vi "test_MSS simulated daqmx do.vi"(8 "Error In":errorcluster) -> (0 "Error Out":errorcluster)   [LabVIEW 2023]
uses:
  Virtual DIO/Virt PWM Generator/Virt DAQmx PWM Generator.lvclass
  Measure and Stimulus Subsystems/Measure and Stimulus Subsystems.lvclass
panel:
  in  "Stop":bool
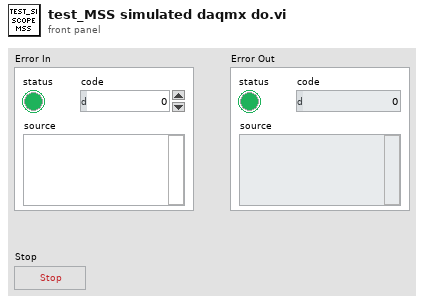
[diagram p1: front panel]
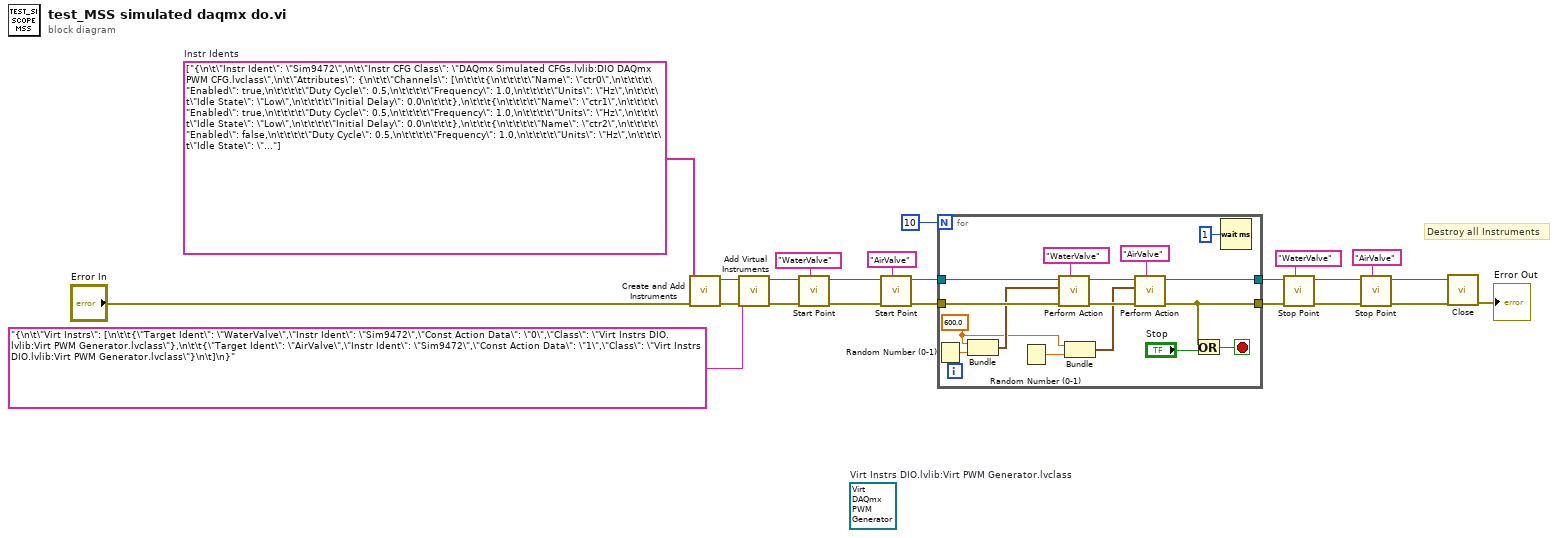
[diagram p0: block diagram]
diagram:
  (unwired) refnum<class "Virt DAQmx PWM Generator.lvclass"> refnum  # Virt Instrs DIO.lvlib:Virt PWM Generator.lvclass
  w19 = string[] ["{\n\t\"Instr Ident\": \"Sim9472\",\n\t\"Instr CFG Class\": \"DAQmx Simulated CFGs.lvlib:DIO DAQmx PWM CFG.lvclass\",\n\t\"Attributes\": {\n\t\t\"Channels\": [\n\t\t\t{\n\t\t\t\t\"Name\": \"ctr0\",\n\t\t\t\t\"Enabled\": true,\n\t\t\t\t\"Duty Cycle\": 0.5,\n\t\t\t\t\"Frequency\": 1.0,\n\t\t\t\t\"Units\": \"Hz\",\n\t\t\t\t\"Idle State\": \"Low\",\n\t\t\t\t\"Initial Delay\": 0.0\n\t\t\t},\n\t\t\t{\n\t\t\t\t\"Name\": \"ctr1\",\n\t\t\t\t\"Enabled\": true,\n\t\t\t\t\"Duty Cycle\": 0.5,\n\t\t\t\t\"Frequency\": 1.0,\n\t\t\t\t\"Units\": \"Hz\",\n\t\t\t\t\"Idle State\": \"Low\",\n\t\t\t\t\"Initial Delay\": 0.0\n\t\t\t},\n\t\t\t{\n\t\t\t\t\"Name\": \"ctr2\",\n\t\t\t\t\"Enabled\": false,\n\t\t\t\t\"Duty Cycle\": 0.5,\n\t\t\t\t\"Frequency\": 1.0,\n\t\t\t\t\"Units\": \"Hz\",\n\t\t\t\t\"Idle State\": \"Low\",\n\t\t\t\t\"Initial Delay\": 0.0\n\t\t\t},\n\t\t\t{\n\t\t\t\t\"Name\": \"ctr3\",\n\t\t\t\t\"Enabled\": false,\n\t\t\t\t\"Duty Cycle\": 0.5,\n\t\t\t\t\"Frequency\": 1.0,\n\t\t\t\t\"Units\": \"Hz\",\n\t\t\t\t\"Idle State\": \"Low\",\n\t\t\t\t\"Initial Delay\": 0.0\n\t\t\t}\n\t\t],\n\t\t\"Timing\": {\n\t\t\t\"Samples per Channel\": 1000,\n\t\t\t\"Sample Mode\": \"Continuous Samples\",\n\t\t\t\"Sample Rate\": 0.0,\n\t\t\t\"Sample Clock Source\": \"Implicit\",\n\t\t\t\"Active Edge\": \"Rising\"\n\t\t},\n\t\t\"Trigger\": {\n\t\t\t\"Trigger Type\": \"No Trigger\"\n\t\t}\n\t}\n}"]  # Instr Idents
  # "Destroy all Instruments"
  n1 = call "Create and Add Instruments.vi"("Error In"="Error In", "Physical Intr CFGs"=w19) -> ("Error Out"=w20:errorcluster, "MSS out"=w5:refnum<class "Measure and Stimulus Subsystems.lvclass">)  [unwired: 8 in]
  n2 = call "Add Virtual Instruments.vi"("error in"=w20, "<JSON CFG>"="{\n\t\"Virt Instrs\": [\n\t\t{\"Target Ident\": \"WaterValve\",\"Instr Ident\": \"Sim9472\",\"Const Action Data\": \"0\",\"Class\": \"Virt Instrs DIO.lvlib:Virt PWM Generator.lvclass\"},\n\t\t{\"Target Ident\": \"AirValve\",\"Instr Ident\": \"Sim9472\",\"Const Action Data\": \"1\",\"Class\": \"Virt Instrs DIO.lvlib:Virt PWM Generator.lvclass\"}\n\t]\n}", "MSS in"=w5) -> ("error out"=w6:errorcluster, "MSS out"=w4:refnum<class "Measure and Stimulus Subsystems.lvclass">)  [unwired: 7 in]
  n3 = call "Start Point.vi"("Point Ident"="WaterValve" ("Target Ident"), "error in"=w6, "MSS in"=w4) -> ("error out"=w18:errorcluster, "MSS out"=w16:refnum<class "Measure and Stimulus Subsystems.lvclass">)  [unwired: 7 in]
  n4 = call "Start Point.vi"("Point Ident"="AirValve" ("Target Ident"), "error in"=w18, "MSS in"=w16) -> ("error out"=w17:errorcluster, "MSS out"=w15:refnum<class "Measure and Stimulus Subsystems.lvclass">)  [unwired: 7 in]
  n5 = for {
    N: 10 -> [_]
    tunnel: w17 -> [w34]
    tunnel: w15 -> [w33]
    tunnel: [w35] -> w11
    tunnel: [w37] -> w22
    stop <- w39 stop-if-true
    w25 = 600.0
    n6 = Random Number (0-1)() -> (number: 0 to 1=w29:dbl)
    n7 = Bundle(w25, "number: 0 to 1"=w29) -> (w26:cluster{dbl, "number: 0 to 1":dbl})  [unwired: 1 in]
    n8 = Random Number (0-1)() -> (number: 0 to 1=w28:dbl)
    n9 = call "Perform Action.vi"("Point Ident"="WaterValve" ("Target Identifier"), "error in"=w34, "Input"=w26, "MSS in"=w33) -> ("error out"=w32:errorcluster, "MSS out"=w30:refnum<class "Measure and Stimulus Subsystems.lvclass">)  [unwired: 5 in, 1 out]
    n10 = Bundle(w25, "number: 0 to 1"=w28) -> (w27:cluster{dbl, "number: 0 to 1":dbl})  [unwired: 1 in]
    n11 = call "Perform Action.vi"("Point Ident"="AirValve" ("Target Identifier"), "error in"=w32, "Input"=w27, "MSS in"=w30) -> ("error out"=w37:errorcluster, "MSS out"=w35:refnum<class "Measure and Stimulus Subsystems.lvclass">)  [unwired: 5 in, 1 out]
    n12 = Or(x=w37, y="Stop") -> (x .or. y?=w39:bool)
    n13 = Wait (ms)(milliseconds to wait=u32 1) -> ()  [unwired: 1 out]
  }
  n14 = call "Stop Point.vi"("Point Ident"="WaterValve" ("Target Ident"), "error in"=w22, "MSS in"=w11) -> ("error out"=w12:errorcluster, "MSS out"=w10:refnum<class "Measure and Stimulus Subsystems.lvclass">)  [unwired: 7 in]
  n15 = call "Stop Point.vi"("Point Ident"="AirValve" ("Target Ident"), "error in"=w12, "MSS in"=w10) -> ("error out"=w1:errorcluster, "MSS out"=w2:refnum<class "Measure and Stimulus Subsystems.lvclass">)  [unwired: 7 in]
  n16 = call "Close.vi"("error in"=w1, "MSS in"=w2) -> ("error out"=→"Error Out":errorcluster)  [unwired: 8 in, 1 out]
